vi "AggregateResults (Variant Map).vi"(7 "Section":string, 8 "error in (no error)":errorcluster, 10 "Results":map{string, variant}(c390), 11 "Pips in":refnum<class "Pips.lvclass">) -> (0 "error out":errorcluster, 3 "Pips out":refnum<class "Pips.lvclass">)   [LabVIEW 2021, in "Bananas.lvlib" / "Pips.lvclass"]
uses:
  Pips.lvclass
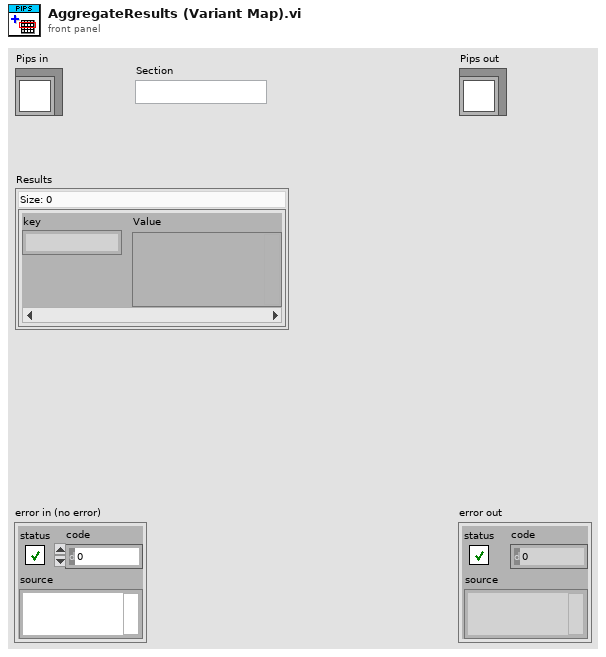
[diagram p1: front panel]
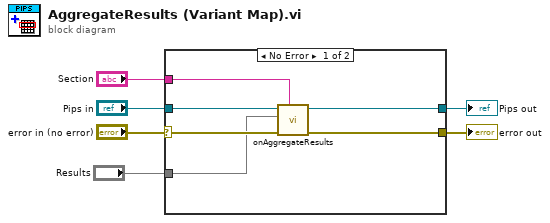
[diagram p0: block diagram]
diagram:
  n1 = case shown="No Error" "error in (no error)" {
    selector: "error in (no error)" -> [w9 w14]
    tunnel: [w10 w14] -> w5
    tunnel: [w11 w13] -> w3
    tunnel: "Pips in" -> [w12 w13]
    tunnel: "Results" -> [w8 _]
    tunnel: "Section" -> [w7 _]
    frame No Error {
      n2 = call-dynamic "onAggregateResults.vi"("Section"=w7, "error in (no error)"=w9, "Results"=w8, "Pips in"=w12) -> ("error out"=w10:errorcluster, "Pips out"=w11:refnum<class "Pips.lvclass">)  [unwired: 6 in]
    }
    frame Error {
    }
  }
  "error out" <- w5
  "Pips out" <- w3
